vi "Robot Info Loop.vi"   [LabVIEW 2016]
uses:
  Common Code/Robot Status Cluster.ctl
  <vilib>/Rock Robotics/WPI/DriverStation/WPI_DriverStationRobotMode2.ctl
  <vilib>/Rock Robotics/WPI/DriverStation/WPI_DriverStationAllianceInfo.ctl
  <vilib>/Rock Robotics/WPI/DriverStation/WPI_DriverStationPositionInfo.ctl
  Robot Global Data.vi
types:
  T1 = typedef "Robot Status Cluster.ctl" = cluster{"RobotMode":T2, "Alliance":T3, "Position":T4, "Match Time":dbl, "FMS?":bool}
  T2 = typedef "WPI_DriverStationRobotMode2.ctl" = enum16{"Autonomous Disabled", "Autonomous Enabled", "Teleop Disabled", "Teleop Enabled", "Disconnected", "Finish", "Test Disabled", "Test Enabled", "Emergency Stopped"}
  T3 = typedef "WPI_DriverStationAllianceInfo.ctl" = enum16{"Red", "Blue", "Invalid"}
  T4 = typedef "WPI_DriverStationPositionInfo.ctl" = enum16{"1", "2", "3"}
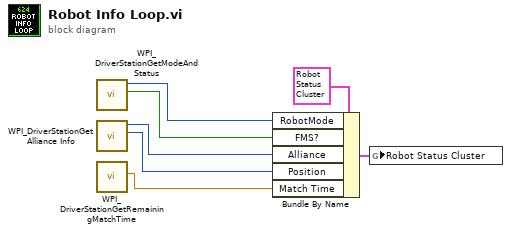
[diagram p0: block diagram]
diagram:
  n1 = call <vilib>:"WPI_DriverStationGetModeAndStatus.vi"() -> ("FMS Attached"=w1:bool, "Robot Mode"=w2:T2)  [unwired: 10 in]
  n2 = call <vilib>:"WPI_DriverStationGet Alliance Info.vi"() -> ("Position"=w3:T4, "Alliance"=w4:T3)  [unwired: 10 in]
  n3 = call <vilib>:"WPI_DriverStationGetRemainingMatchTime.vi"() -> ("Match Time(s)"=w5:sgl)  [unwired: 10 in, 1 out]
  n4 = Bundle By Name(cluster=T1 {"RobotMode"=enum."Autonomous Disabled", "Alliance"=enum."Red", "Position"=enum."1", "Match Time"=0.0, "FMS?"=FALSE} ("Robot Status Cluster"), "RobotMode"=w2, "FMS?"=w1, "Alliance"=w4, "Position"=w3, "Match Time"=w5) -> (w6:T1)
  n5 = global write "Robot Global Data.vi" "Robot Status Cluster"(w6) -> ()
